vi "MHM Set Interface.vi"(8 "error in (no error)":errorcluster, 9 "pcInterfaceOption":string, 10 "ulInterface":u32, 11 "ulMHMHandle":u32) -> (0 "error out":errorcluster, 3 "function return":u32)   [LabVIEW 2017, in "MHM_1SL_interface.lvlib"]
uses:
  MHM_1SL_interface.lvlib
  lib/MHM_1SL_interface.dll
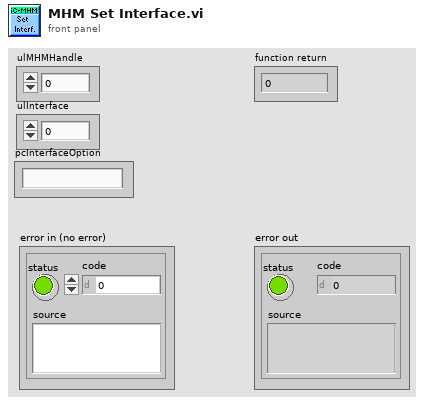
[diagram p1: front panel]
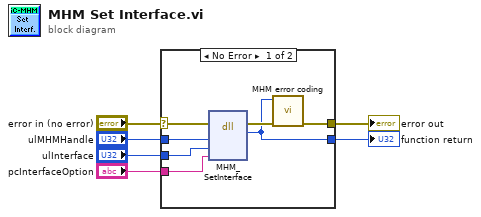
[diagram p0: block diagram]
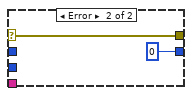
[diagram p2: hidden frame]
diagram:
  n1 = case shown="No Error" "error in (no error)" {
    selector: "error in (no error)" -> [w13 w15]
    tunnel: "ulMHMHandle" -> [w12 _]
    tunnel: "ulInterface" -> [w11 _]
    tunnel: [w9 w15] -> w3
    tunnel: [w8 u32 0] -> w2
    tunnel: "pcInterfaceOption" -> [w7 _]
    frame No Error {
      n2 = dll-call lib="C:/workspace/project/scancon/sw/SSI_Tool/DUT_Interface/lv_interface/lib/MHM_1SL_interface.dll" fn="MHM_SetInterface"(error in=w13, "ulMHMHandle"=w12, "ulInterface"=w11, "pcInterfaceOption"=w7) -> (error out=w10:errorcluster, "return type"=w8:u32)  [unwired: 5 in, 1 out]
      n3 = call "MHM error coding.vi"("error in (no error)"=w10, "function return in"=w8) -> ("error out"=w9:errorcluster)  [unwired: 9 in]
    }
    frame Error {
    }
  }
  "function return" <- w2
  "error out" <- w3
